vi "Open and Setup CAN Session.vi"(8 "error in":errorcluster, 11 "measurement configuration":T1 {"Baudrate" format="%x"; "FD Baudrate" format="%x"}) -> (0 "error out":errorcluster, 2 "session out":refnum<k21>)   [LabVIEW 2025, in "CAN-LIN Raw Bus Capture.lvclass"]
uses:
  CAN-LIN Raw Bus Capture.lvclass
  Measurement Configuration.ctl
  CAN-LIN Raw Bus Capture UI/Toggle.ctl
  <vilib>/xnet/xnet.llb/XNET Create Session (Frame Input Stream).vi
  CAN-LIN Raw Bus Capture.lvclass/CAN-LIN Raw Bus Capture.ctl
  <resource>/objmgr/xnet.rc
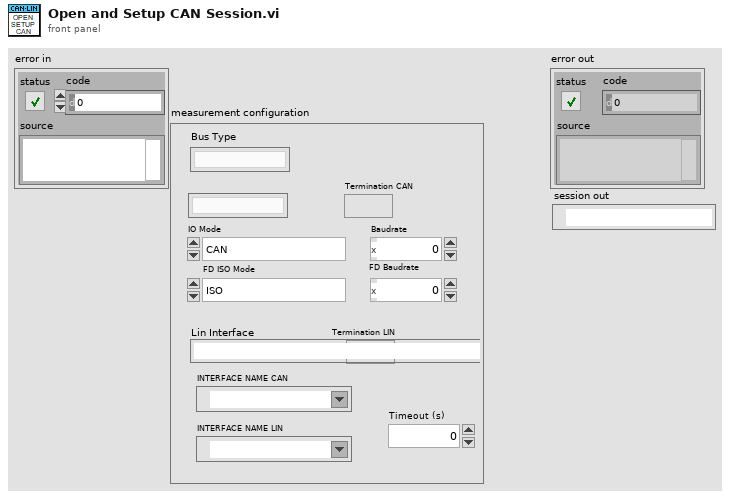
[diagram p1: front panel]
types:
  T1 = typedef "CAN-LIN Raw Bus Capture.lvclass/Measurement Configuration.ctl" = cluster{"Termination CAN":T2, "FD Baudrate":u32, "Baudrate":u32, "FD ISO Mode":enum32{"ISO", "Legacy ISO", "Non-ISO"}, "IO Mode":enum32{"CAN", "CAN FD", "CAN FD + BRS"}, "Termination LIN":T2, "Can Interface":string, "Lin Interface":string, "Bus Type":string, "INTERFACE NAME CAN":refnum<k21>, "INTERFACE NAME LIN":refnum<k21>, "Timeout (s)":u32}
  T2 = typedef "Toggle.ctl" = bool
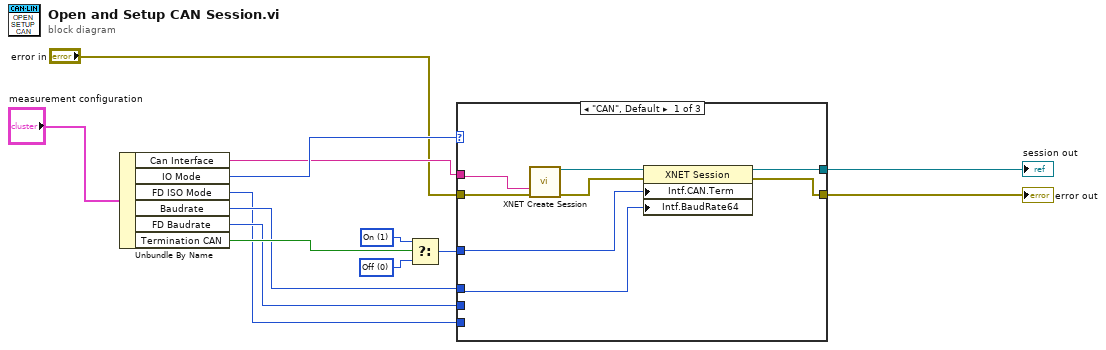
[diagram p0: block diagram]
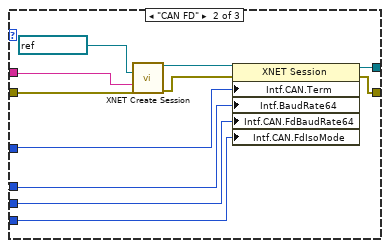
[diagram p2: hidden frame]
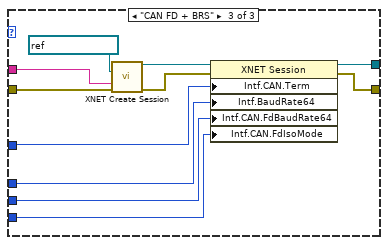
[diagram p3: hidden frame]
diagram:
  w11 = u32 1 items=["Off", "On"] ("Interface:CAN:Termination")
  w12 = u32 0 items=["Off", "On"] ("Interface:CAN:Termination")
  n1 = Unbundle By Name("measurement configuration") -> ("Can Interface"=w5:string, "IO Mode"=w10:enum32{"CAN", "CAN FD", "CAN FD + BRS"}, "FD ISO Mode"=w6:enum32{"ISO", "Legacy ISO", "Non-ISO"}, "Baudrate"=w8:u32, "FD Baudrate"=w7:u32, "Termination CAN"=w13:T2)
  n2 = Select(t=w11, s=w13, f=w12) -> (s? t:f=w9:u32)
  n3 = case shown="\"CAN\", Default" w10 {
    tunnel: [w19 w25 w40] -> w1
    tunnel: w5 -> [w16 w29 w36]
    tunnel: "error in" -> [w18 w28 w35]
    tunnel: [w17 w24 w33] -> w2
    tunnel: w8 -> [w14 w27 w39]
    tunnel: w7 -> [_ w23 w38]
    tunnel: w6 -> [_ w26 w37]
    tunnel: w9 -> [w15 w22 w34]
    frame "CAN", Default {
      n4 = call-poly <vilib>:"XNET Create Session.vi"("interface"=w16, "error in (no error)"=w18) -> ("session out"=w21:refnum<k21>, "error out"=w20:errorcluster)  [unwired: 12 in]
      n5 = property class="XNET Session"(reference=w21, error in=w20, "Intf.CAN.Term"=w15, "Intf.BaudRate64"=w14) -> (reference out=w19:refnum<k21>, error out=w17:errorcluster)
    }
    frame "CAN FD" {
      n6 = call-poly <vilib>:"XNET Create Session.vi"("cluster (:memory:)"=refnum<k21> ":can_fd:", "interface"=w29, "error in (no error)"=w28) -> ("session out"=w31:refnum<k21>, "error out"=w30:errorcluster)  [unwired: 11 in]
      n7 = property class="XNET Session"(reference=w31, error in=w30, "Intf.CAN.Term"=w22, "Intf.BaudRate64"=w27, "Intf.CAN.FdBaudRate64"=w23, "Intf.CAN.FdIsoMode"=w26) -> (reference out=w25:refnum<k21>, error out=w24:errorcluster)
    }
    frame "CAN FD + BRS" {
      n8 = call-poly <vilib>:"XNET Create Session.vi"("cluster (:memory:)"=refnum<k21> ":can_fd_brs:", "interface"=w36, "error in (no error)"=w35) -> ("session out"=w42:refnum<k21>, "error out"=w41:errorcluster)  [unwired: 11 in]
      n9 = property class="XNET Session"(reference=w42, error in=w41, "Intf.CAN.Term"=w34, "Intf.BaudRate64"=w39, "Intf.CAN.FdBaudRate64"=w38, "Intf.CAN.FdIsoMode"=w37) -> (reference out=w40:refnum<k21>, error out=w33:errorcluster)
    }
  }
  "error out" <- w2
  "session out" <- w1
